vi "Time_Trace_File_to_Clusters.vi"(11 "selected path":path) -> (2 "Analysis Info Cluster Array":T2[](array[typedef]) {"Kurt_u" format="%_3g"; "u^4" format="%_3g"; "u^3" format="%_3g"; "Sd Error in Variance" format="%_3g"; "u^2" format="%_3g"; "Sd Error in Mean" format="%_3g"; "U" format="%_3g"; "Sync Delay Time (s)" format="%.4f"; "Total Meas Time (s)" format="%_5g"; "Skew_u" format="%_3g"; "% u'/U" format="%_3g"}, 3 "Time Trace Cluster Array":T1[](array[typedef]), 5 "times":dbl[](array[numeric]))   [LabVIEW 2022 SP3]
uses:
  Data_plotting_vis/Data_File_Type.ctl
  Controls/Time_Trace_Cluster.ctl
  Controls/Instrument_Array.ctl
  Controls/Inst_type.ctl
  Controls/Analysis_info_cluster.ctl
  Controls/channelState.ctl
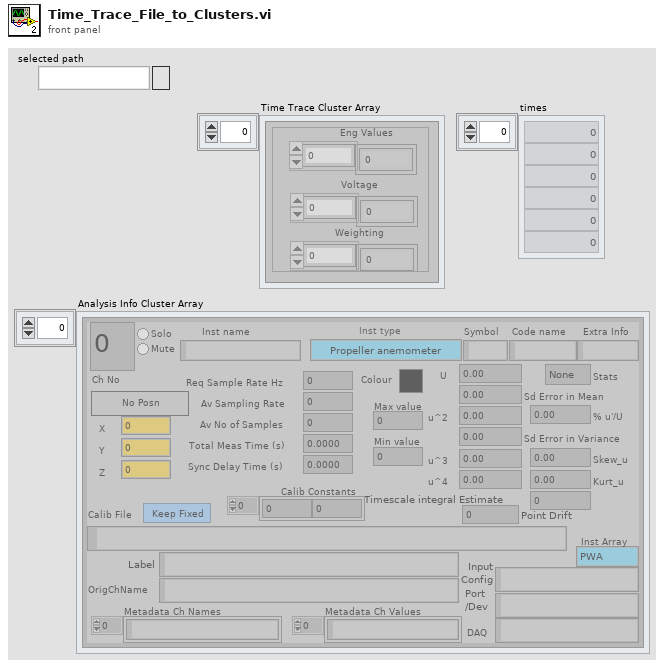
[diagram p1: front panel]
types:
  T1 = typedef "Time_Trace_Cluster.ctl" = cluster{"Weighting":dbl[], "Voltage":dbl[], "Eng Values":dbl[]}
  T2 = typedef "Analysis_info_cluster.ctl" = cluster{"Colour":u32, "Inst type":T3, "Inst name":string, "Symbol":string, "Code name":string, "Extra Info":string, "Inst Array":T4, "U":dbl, "u^2":dbl, "u^3":dbl, "u^4":dbl, "Skew_u":dbl, "Kurt_u":dbl, "Sd Error in Mean":dbl, "% u'/U":dbl, "X":dbl, "Y":dbl, "Z":dbl, "Timescale integral Estimate":dbl, "Sd Error in Variance":dbl, "Calib File":path, "Calib Constants":dbl[], "Output Position":bool, "Stats":enum16{"None", "Basic", "Full"}, "Av Sampling Rate":dbl, "Av No of Samples":dbl, "Total Meas Time (s)":dbl, "OrigChName":string, "Max value":dbl, "Min value":dbl, "Req Sample Rate Hz":dbl, "Sync Delay Time (s)":dbl, "Ch No":i16, "Device":string, "Use Latest Calib":bool, "Port":string, "Metadata Ch Names":string[], "Metadata Ch Values":string[], "Label":string, "chState":T5, "Point Drift":dbl, "inputConfig":string}
  T3 = typedef "Inst_type.ctl" = enum16{"Raw voltage", "Raw with zero offsetting", "Propeller anemometer", "Pressure Transducer", "Pitot-static tube", "Hot wire", "Cross wire 1", "Cross wire 2", "Generic Linear", "Generic Polynomial", "Generic BackPoly", "Fast FID", "Thermocouple", "Cold wire", "Pulsed Wire", "LDA Vel", "LDA Tran time", "LDA Arr time", "Microphone"}
  T4 = typedef "Instrument_Array.ctl" = enum16{"PWA", "LDA", "Analogue"}
  T5 = typedef "channelState.ctl" = enum32{"No Selection", "Solo", "Mute"}
  T6 = typedef "Data_File_Type.ctl" = enum16{"Read All File Types", "Results Files Only", "Raw Data Files Only", "Calibration Files Only", "Gas Desk Files Only", "Old Results Files Only", "Tabulated Data Files Only"}
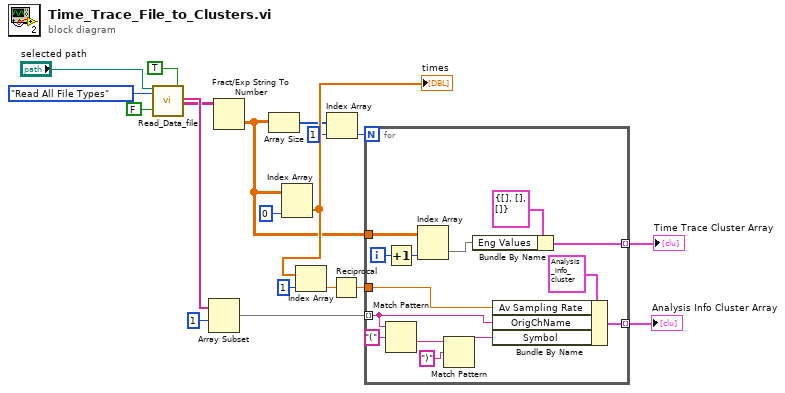
[diagram p0: block diagram]
diagram:
  n1 = call "Read_Data_file.vi"("Results file"="selected path", "Delete First Rows?"=TRUE, "Run EnFlo Hub? (T)"=FALSE, "Desired File Types"=Data_File_Type."Read All File Types") -> ("Ch names Out"=w13:string[], "Channel Values Out"=w6:string[][])  [unwired: 6 in, 8 out]
  n2 = Array Subset(array=w13, index=1) -> (w15:string[])  [unwired: 1 in]
  n3 = Fract/Exp String To Number(string=w6) -> (number=w11:dbl[][])  [unwired: 3 in, 1 out]
  n4 = Array Size(array=w11) -> (size(s)=w9:i32[])
  n5 = Index Array(array=w11, index (col)=0 ("disabled index (col)")) -> (element=w19:dbl[])  [unwired: 1 in]
  "times" <- w19
  n6 = Index Array(array=w19, index=1) -> (element=w2:dbl)
  n7 = Index Array(array=w9, index=1 ("index (row)")) -> (element=w10:i32)
  n8 = Reciprocal(x=w2) -> (1/x=w1:dbl)
  n9 = for {
    N: w10 -> [_]
    tunnel: [w32] -> w12 mode=indexing
    tunnel: w11 -> [w29]
    tunnel: w15 -> [w20] mode=indexing
    tunnel: [w26] -> w16 mode=indexing
    tunnel: w1 -> [w22]
    i -> [w30]
    n10 = Increment(x=w30) -> (x+1=w31:i32)
    n11 = Match Pattern(string=w20, regular expression="(") -> (after substring=w24:string)  [unwired: 1 in, 3 out]
    n12 = Index Array(array=w29, index (col)=w31) -> (element=w28:dbl[])  [unwired: 1 in]
    n13 = Match Pattern(string=w24, regular expression=")") -> (before substring=w21:string)  [unwired: 1 in, 3 out]
    n14 = Bundle By Name(cluster=T1 {"Weighting"=[], "Voltage"=[], "Eng Values"=[]} ("Time Trace"), "Eng Values"=w28) -> (w32:T1)
    n15 = Bundle By Name(cluster=T2 {"Colour"=0, "Inst type"=enum."Pitot-static tube", "Inst name"="Manometer voltage", "Symbol"="U", "Code name"="", "Extra Info"="U", "Inst Array"=enum."PWA", "U"=0.0, "u^2"=0.0, "u^3"=0.0, "u^4"=0.0, "Skew_u"=0.0, "Kurt_u"=0.0, "Sd Error in Mean"=0.0, "% u'/U"=0.0, "X"=0.0, "Y"=0.0, "Z"=0.0, "Timescale integral Estimate"=0.0, "Sd Error in Variance"=0.0, "Calib File"=path "", "Calib Constants"=[], "Output Position"=FALSE, "Stats"=enum."None", "Av Sampling Rate"=0.0, "Av No of Samples"=0.0, "Total Meas Time (s)"=0.0, "OrigChName"="", "Max value"=0.0, "Min value"=0.0, "Req Sample Rate Hz"=0.0, "Sync Delay Time (s)"=0.0, "Ch No"=0, "Device"="", "Use Latest Calib"=FALSE, "Port"="", "Metadata Ch Names"=[], "Metadata Ch Values"=[], "Label"="", "chState"=enum."No Selection", "Point Drift"=0.0, "inputConfig"=""}, "Av Sampling Rate"=w22, "OrigChName"=w20, "Symbol"=w21) -> (w26:T2)
  }
  "Analysis Info Cluster Array" <- w16
  "Time Trace Cluster Array" <- w12
